vi "Initialize-cRIO-USB.vi"(5 "Reset? (F: No)":bool, 6 "Checksum (Disabled)":bool, 7 "ID Query? (Enabled)":bool=TRUE, 8 "error in (no error)":errorcluster, 10 "Protocol (2: SCIP 2.0)":u32(ring)=2 items=["Convert to Latest", "SCIP 1.1", "SCIP 2.0"], 11 "VISA resource name":refnum<visa-resource-name>) -> (0 "error out":errorcluster, 3 "VISA resource name out":refnum<visa-resource-name>)   [LabVIEW 2011, in "Hokuyo URG Series.lvlib"]
doc: "Establishes communication with the instrument. It also places the instrument in a default state needed for other instrument driver operations. Therefore, call this VI before calling other instrument driver VIs for this instrument. Generally, you need to call the Initialize VI only once at the beginning of an application.\n\n<b>Note:</b> This VI is meant to be used when controlling the instrument from an NI Compact RIO USB port."
uses:
  Hokuyo URG Series.lvlib
panel:
  # "(c) 2009 National Instruments.  ALL RIGHTS RESERVED."
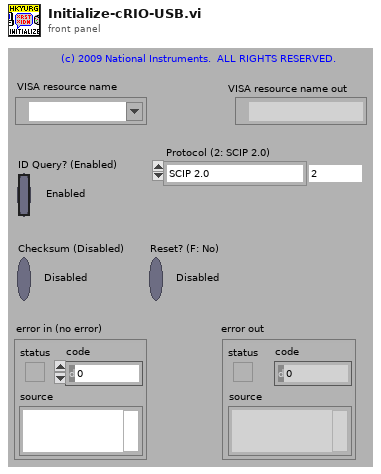
[diagram p1: front panel]
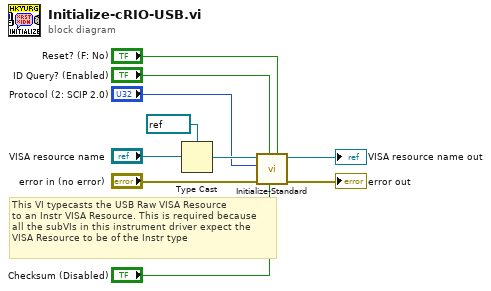
[diagram p0: block diagram]
diagram:
  # "This VI typecasts the USB Raw VISA Resource\nto an Instr VISA Resource. This is required because\nall the subVIs in this instrument driver expect the\nVISA Resource to be of the Instr type"
  n1 = Type Cast(type=refnum<visa-resource-name> refnum ("VISA resource name out"), x="VISA resource name") -> (*(type *) &x=w4:refnum<visa-resource-name>)
  n2 = call "Initialize-Standard.vi"("Reset? (F: No)"="Reset? (F: No)", "Checksum (Disabled)"="Checksum (Disabled)", "ID Query? (Enabled)"="ID Query? (Enabled)", "error in (no error)"="error in (no error)", "Protocol (2: SCIP 2.0)"="Protocol (2: SCIP 2.0)", "VISA resource name"=w4) -> ("error out"=→"error out":errorcluster, "VISA resource name out"=→"VISA resource name out":refnum<visa-resource-name>)  [unwired: 4 in]
